vi "Lvi Subsystem Properties.vi"(8 "error in (no error)":errorcluster, 9 "CapNumber":u32, 10 "EnumCap":u32, 11 "TaskRef":i32) -> (0 "error out":errorcluster, 1 "ValueOne":dbl, 2 "NumCapsFound":u32, 3 "TaskRef out":i32, 4 "function return":u32(ring), 5 "ValueTwo":dbl)   [LabVIEW 2022 SP3, in "DtLvLink.lvlib"]
doc: "Calls directly into the entry points of the DLL of the Data Acq SDK to configure the specified task. This VI is used by the higher-level VI, DtOLSubsystem."
uses:
  DtLvLink.lvlib
  <userlib>/LV-Link3/DtLvLink_64.dll
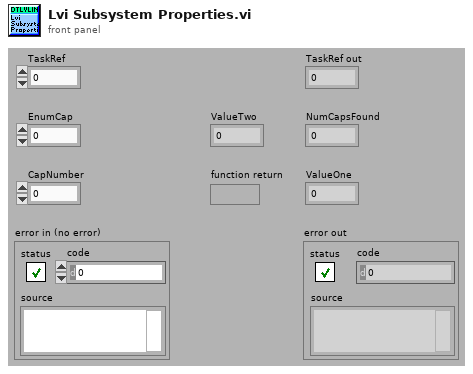
[diagram p1: front panel]
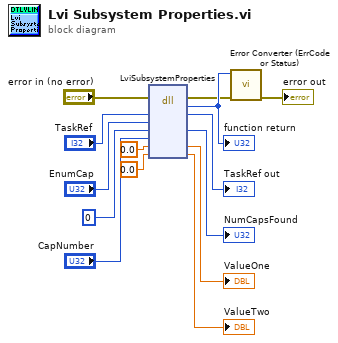
[diagram p0: block diagram]
diagram:
  n1 = dll-call lib="C:/Program Files/National Instruments/LabVIEW 2022/user.lib/LV-Link3/DtLvLink_64.*" fn="LviSubsystemProperties"(error in="error in (no error)", "TaskRef"="TaskRef", "EnumCap"="EnumCap", "NumCapsFound"=u32 0, "CapNumber"="CapNumber", "ValueOne"=0.0, "ValueTwo"=0.0) -> (error out=w2:errorcluster, w14:u32, "TaskRef"=→"TaskRef out":i32, "NumCapsFound"=→"NumCapsFound":u32, "ValueOne"=→"ValueOne":dbl, "ValueTwo"=→"ValueTwo":dbl)  [unwired: 4 in, 1 out]
  "function return" <- w14
  n2 = call "Error Converter (ErrCode or Status).vi"("error in (no error)"=w2, "error code"=w14) -> ("error out"=→"error out":errorcluster)  [unwired: 9 in]
